vi "Front Panel.vi"(11 "GUI In":refnum<class "Calibration UI.lvclass">) -> ()   [LabVIEW 2015, in "Calibration UI.lvclass"]
uses:
  Calibration UI.lvclass
  Calibration/Collect Data/Collect Data.lvclass
  Calibration/Get Max Orf Flow/Get Max Orifice Flow.lvclass
  Calibration/Set QO2 Rel Flow/Set Rel QO2 flow.lvclass
  Calibration/Set QO2 Rel Flow/Set Rel QO2 flow.lvclass/Set Rel QO2 flow.ctl
  Calibration/Get Max Orf Flow/Get Max Orifice Flow.lvclass/Get Max Orifice Flow.ctl
  Reusable/GUI/GUI.lvclass/GUI.ctl
  Calibration UI.lvclass/Calibration UI.ctl
  Calibration/Collect Data/Collect Data.lvclass/Collect Data.ctl
  Reusable/Sequence/SEQ/SEQ.lvclass
  Reusable/Sequence/STEPS/STEP.lvclass
  Calibration/O3 Generator State/Change O3 Generator State.lvclass
  Calibration/Change Filter State/Change Filter Position.lvclass
  Calibration/Change O2 Valve.lvclass
  Calibration/Wait/Wait.lvclass
  Calibration/Wait/Wait.lvclass/Wait.ctl
  Reusable/Sequence/STEPS/LEAVES/Double/Switch DBL.lvclass/Switch DBL.ctl
  Calibration/O3 Add Valve/Ozone Addition Valve.lvclass
  Calibration/Set O3 Level/Set O3 Level.lvclass
  Calibration/Set O3 Level/Set O3 Level.lvclass/Set O3 Level.ctl
  Calibration/Change Spk Pos/Change Speaker Position.lvclass
  Calibration/State data/State Data.lvclass
  Controls/MFC Address.ctl
  Controls/Flags.ctl
  Reusable/GUI/Accessors/Read RegEvent.vi
  Calibration/Wait/Write Wait Time.vi
  Reusable/Sequence/STEPS/LEAVES/Double/Write val.vi
  Calibration/Collect Data/Write # of Obs.vi
  Calibration/Collect Data/Write Stored State DVR.vi
  Calibration/Collect Data/Write PAS DVR.vi
  Calibration/Collect Data/Write CRD DVR.vi
  Calibration/Collect Data/Write Associated Cells.vi
  Calibration/Set QO2 Rel Flow/Write QO2 DVR.vi
  Calibration/Get Max Orf Flow/Write Max Qorf DVR.vi
panel:
  in  "Lamp":bool
  in  "Lamp Rate (Hz)":i32
  in  "cSequence":bool
  in  "lSequence":bool
  in  "cTable":bool
  out "collPoints":i32
  in  "saveSeq":bool
  in  "Steps":string(tree)
  in  "Sequence":string(tree)
  in  "setCal":bool caption="Set Calibration\nParameters"
  in  "Display":T1(ring)
  in  "O2 Flow":sgl caption="O2 Flow\n(sccm)" format="%.2g"
  in  "Valves":cluster{"O3 Add":bool, "O2 Open":bool}
  out "O3Q":cluster{"Q":sgl, "T":sgl, "P":sgl} caption="Alicat Data" {"P" format="%.2f"; "T" format="%.2f"; "Q" format="%.2f"}
  out "r^2":dbl
  out "Intercept":dbl
  out "Slope":dbl
  out "cal Results":cluster{dbl[], "Upper Bound":dbl[]}[](graph)
  in  "calibrate":bool caption="Run Calibration"
  out "seqMsg":string[](array[string])=["1:09:27 PM\tValve to oxygen changed to TRUE.", "1:09:27 PM\tO2 flow set to 500.000000.", "1:09:32 PM\tMax orifice flow recorded.   Flow was 248.806366.", "1:09:42 PM\tStandard wait time elapsed.", "1:09:54 PM\tStandard wait time elapsed.", "1:09:55 PM\tLaser RMS stable in every cell. RSE Values: 0.000000\t0.000000\r\n", "1:09:55 PM\tSpeaker position changed to TRUE.", "1:09:55 PM\tO2 flow set to 248.806366.", "1:10:01 PM\tOzone stable in every cell.  Begin collecting data. RSE Values: 0.043430\t0.043108\t0.043108\t0.043537\t0.043537\t0.047428\t0.047428\t0.043882\t0.043882\t0.044978\t0.044978\t0.043616\t0.043616\t0.042956\r\n", "1:10:21 PM\tCollection step complete.", "1:10:21 PM\tO2 flow set to 186.604774.", "1:10:27 PM\tOzone stable in every cell.  Begin collecting data. RSE Values: 0.049616\t0.048562\t0.048562\t0.048143\t0.048143\t0.048496\t0.048678\t0.048678\t0.047656\t0.047656\t0.046716\t0.046716\t0.046716\r\n", "1:10:47 PM\tCollection step complete.", "1:10:47 PM\tO2 flow set to 124.403183.", "1:10:53 PM\tOzone stable in every cell.  Begin collecting data. RSE Values: 0.045074\t0.045269\t0.045269\t0.045371\t0.045371\t0.046657\t0.046657\t0.044803\t0.044803\t0.046626\t0.046626\t0.044248\t0.044248\t0.044248\r\n", "1:11:13 PM\tCollection step complete.", "1:11:13 PM\tO2 flow set to 62.201591.", "1:11:19 PM\tOzone stable in every cell.  Begin collecting data. RSE Values: 0.047075\t0.046939\t0.046939\t0.049594\t0.049594\t0.046739\t0.046655\t0.046655\t0.046655\t0.048990\t0.048989\t0.048989\t0.048989\r\n", "1:11:39 PM\tCollection step complete.", "1:11:39 PM\tData displayed!", "1:11:39 PM\tSpeaker position changed to FALSE.", "1:11:39 PM\tValve to oxygen changed to FALSE.", "1:11:39 PM\tO2 flow set to 0.000000.", "1:11:49 PM\tStandard wait time elapsed.", "1:12:02 PM\tStandard wait time elapsed."] caption="Messages"
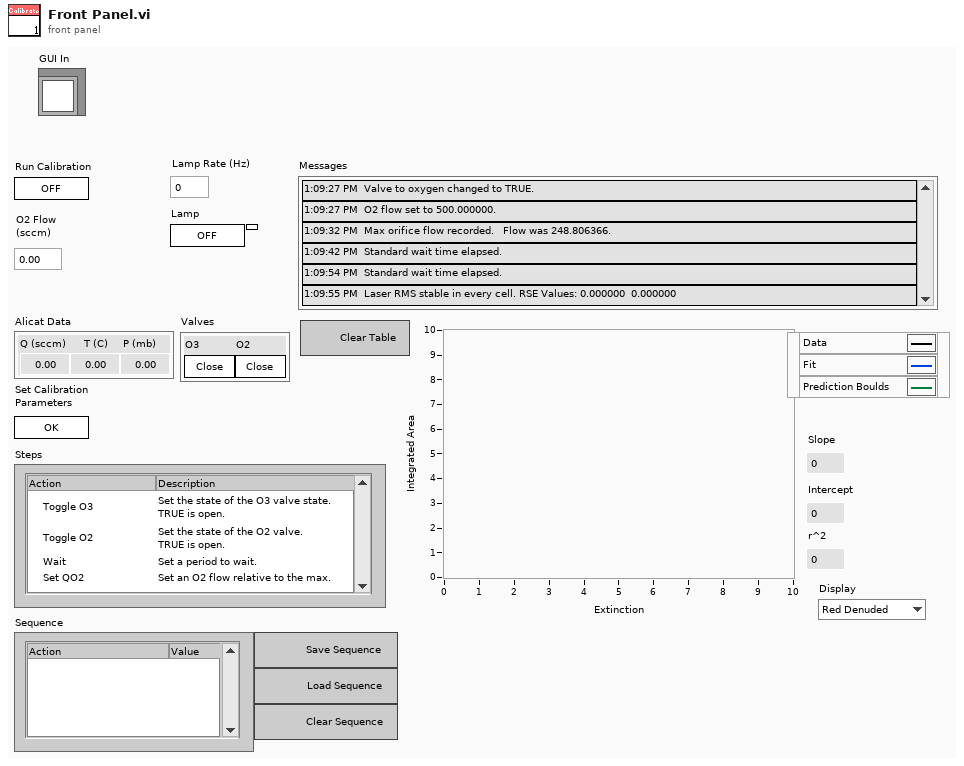
[diagram p1: front panel]
types:
  T1 = enum16{"Red Denuded", "Green", "Red", "Blue", "Blue Denuded"}
  T2 = enum8{"Enabled", "Disabled", "Disabled and Grayed Out"}
  T3 = cluster{"Array of Boolean[0]":bool, "Array of Boolean[1]":bool}
  T4 = cluster{"slope":dbl, "intercept":dbl, "r^2":dbl}[]
  T5 = typedef "Flags.ctl" = enum8{"Autospeaker", "Link cycles", "Autofilter", "O3 Cal", "Filter Position"}
  T6 = typedef "MFC Address.ctl" = enum16{"CRDS Purge", "CRDS Thermodenuded", "CRDS Dry", "CRDS Med RH", "CRDS High RH", "PAS Ch 1", "PAS Ch 2", "PAS Ch3", "PAS Ch 4", "PAS Ch 5", "CLAP", "O3", "Pinlet"}
  T7 = cluster{"Numeric":sgl, "Numeric":sgl, "Numeric":sgl}
  T8 = typedef "eventvkey.ctl" = enum16{"ASCII", "Enter", "Return", "Shift", "Ctrl", "Alt", "Cmd", "Opt", "Caps", "NumLock", "Clear", "Break", "Up", "Down", "Left", "Right", "Insert", "Delete", "Home", "End", "PageUp", "PageDown", "Escape", "Help", "Pause", "ScrollLock", "F1", "F2", "F3", "F4", "F5", "F6", "F7", "F8", "F9", "F10", "F11", "F12", "F13", "F14", "F15", "F16", "F17", "F18", "F19", "F20", "F21", "F22", "F23", "F24", "Play", "VolumeUp", "VolumeDown", "Mute", "Two Byte Char"}
  T9 = cluster{"Stored State":refnum<class "State Data.lvclass">[], "pointer to data":i32}
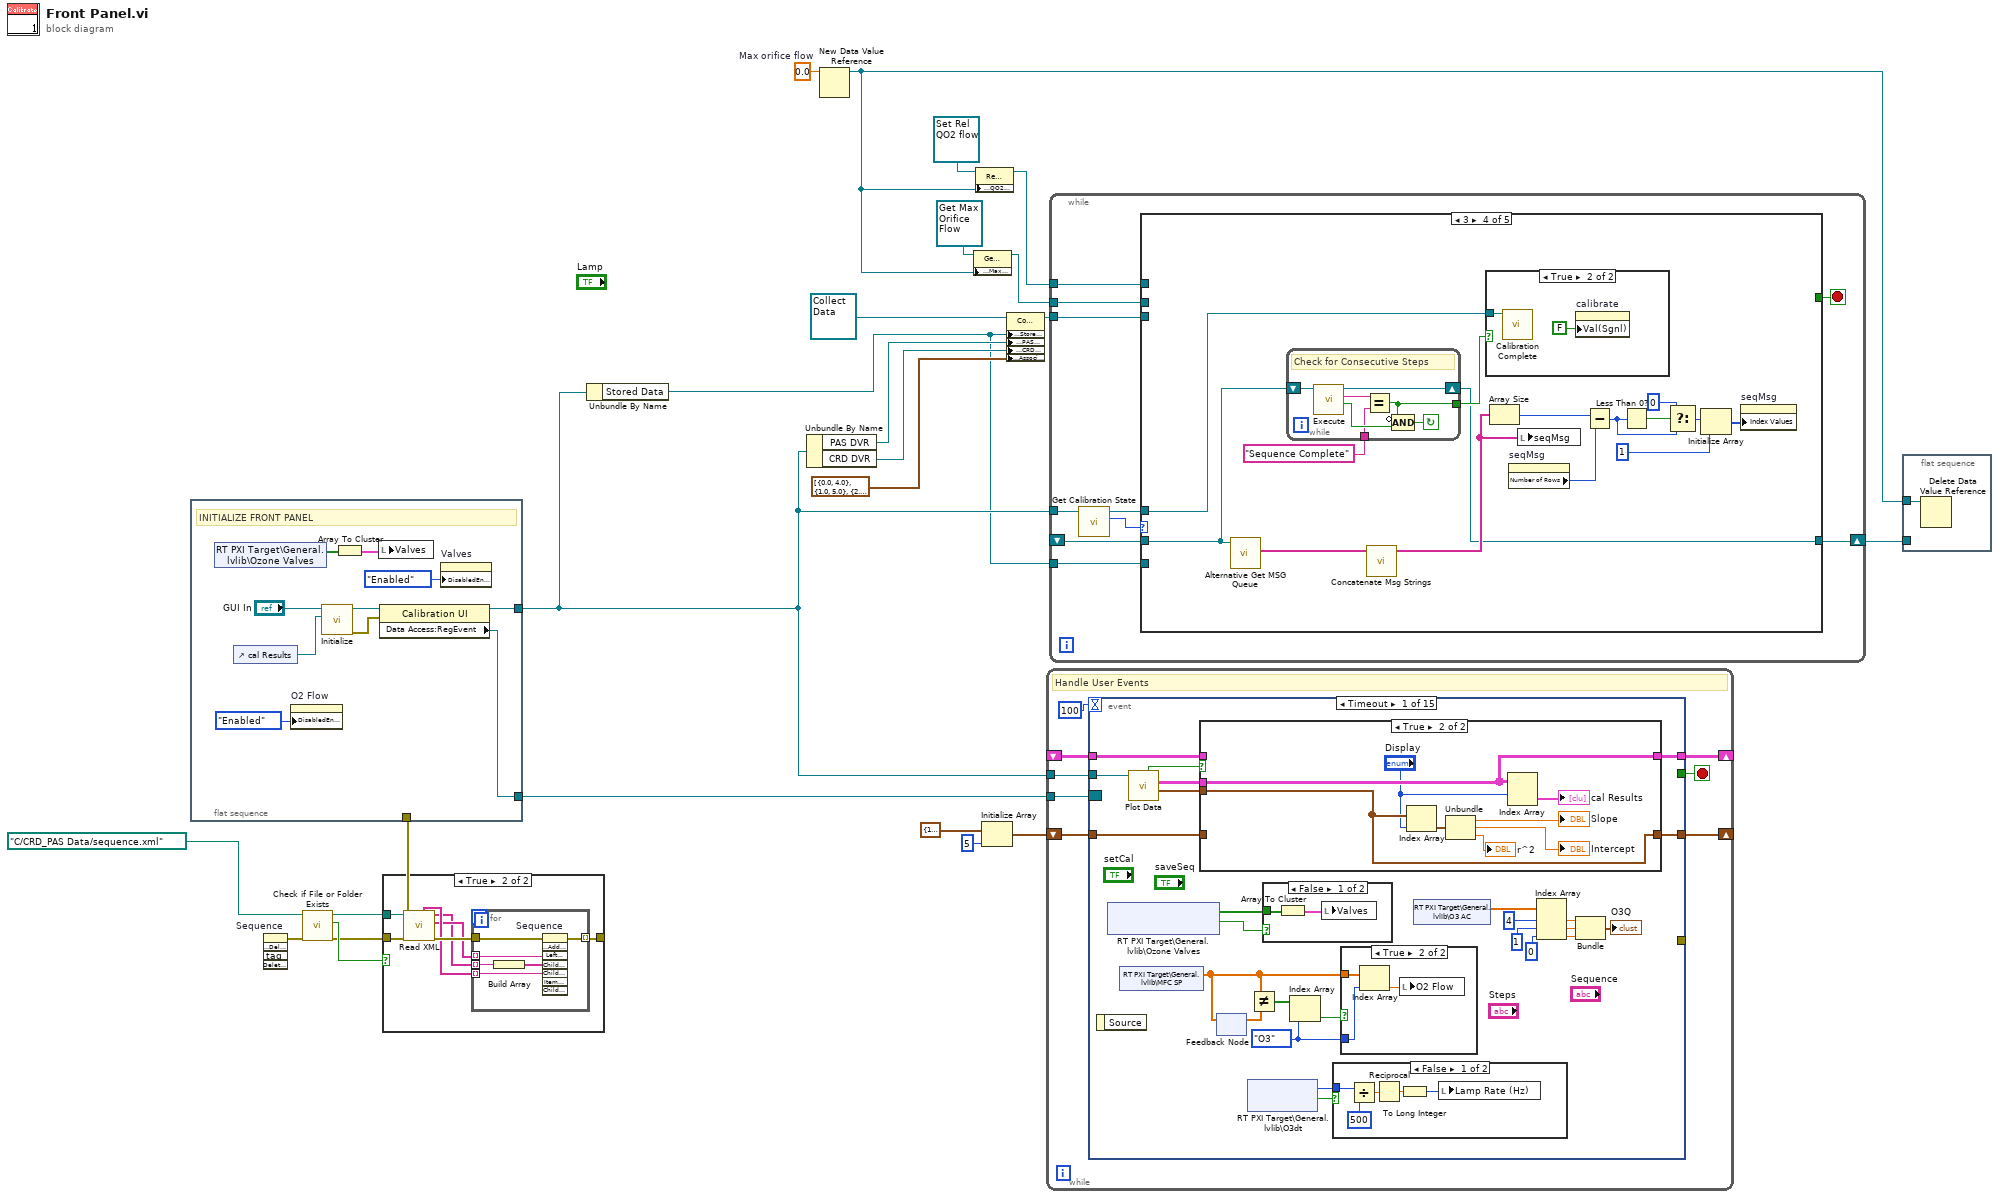
[diagram p0: block diagram]
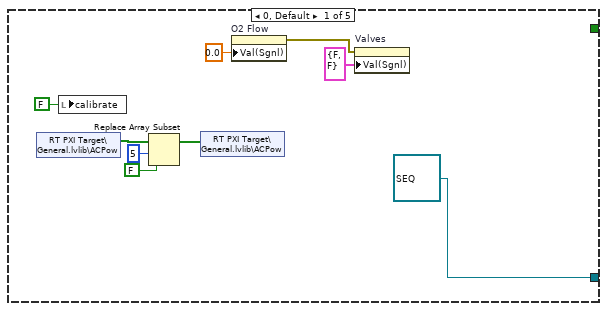
[diagram p3: hidden frame]
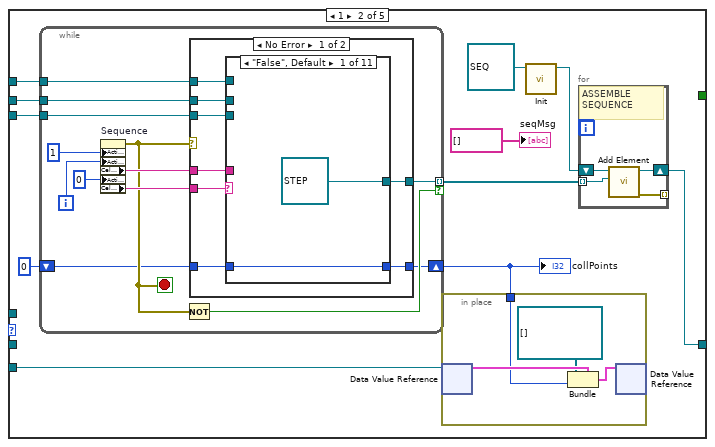
[diagram p4: hidden frame]
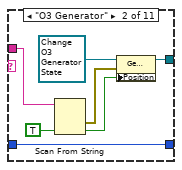
[diagram p5: hidden frame]
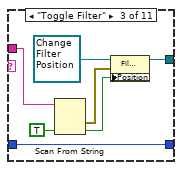
[diagram p6: hidden frame]
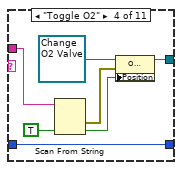
[diagram p7: hidden frame]
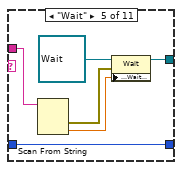
[diagram p8: hidden frame]
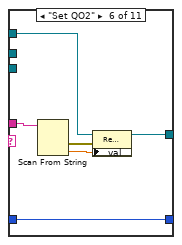
[diagram p9: hidden frame]
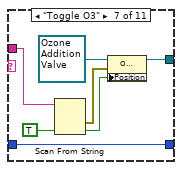
[diagram p10: hidden frame]
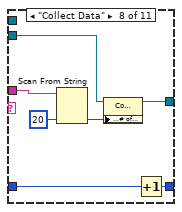
[diagram p11: hidden frame]
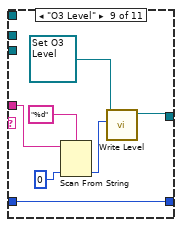
[diagram p12: hidden frame]
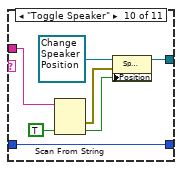
[diagram p13: hidden frame]
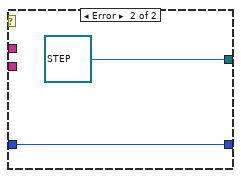
[diagram p15: hidden frame]
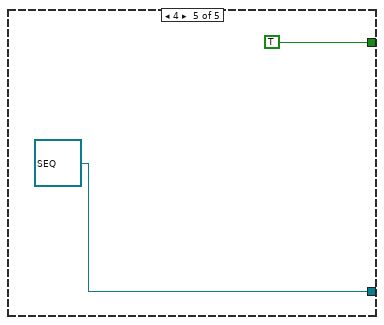
[diagram p18: hidden frame]
diagram:
  w20 = 0.0  # Max orifice flow
  n1 = flat-sequence {
    tunnel: [w27] -> w24
    tunnel: [w26] -> w2
    tunnel: w6 -> [_]
    frame #0 {
      # "INITIALIZE FRONT PANEL"
      n2 = shared-variable "RT PXI Target\\General.lvlib\\Ozone Valves"() -> (w34:bool[])  [unwired: 1 in, 1 out]
      n3 = control-ref of="cal Results"() -> (w30:refnum<vi>)
      n4 = property on="O2 Flow" class="DigNum (strict)"("DisabledEnum"=T2."Enabled" ("Disabled")) -> ()  [unwired: 2 in, 2 out]
      n5 = call "Initialize.vi"("XYGraph in"=w30, "GUI In"="GUI In") -> ("error out"=w29:errorcluster, "GUI Out"=w31:refnum<class "Calibration UI.lvclass">)  [unwired: 8 in]
      n6 = Array To Cluster(array=w34) -> (cluster=w33:T3)
      n7 = local write "Valves"(w33) -> ()
      n8 = property class="Calibration UI"(reference=w31, error in=w29) -> (reference out=w26:refnum<class "Calibration UI.lvclass">, "Data Access:RegEvent"=w27:refnum<event-registration>)  [unwired: 1 out]
      n9 = property on="Valves" class="Clust (strict)"("DisabledEnum"=T2."Enabled" ("Disabled")) -> ()  [unwired: 2 in, 2 out]
    }
  }
  n10 = invoke on="Sequence" class="Tree (strict)" method="Edit Tree Items.Delete"() -> (error out=w9:errorcluster)  [unwired: 5 in, 4 out]
  n11 = call <vilib>:"Check if File or Folder Exists.vi"("error in (no error)"=w9, "path"=path "C:/CRD_PAS Data/sequence.xml" ("file")) -> ("error out"=w8:errorcluster, "file or folder exists?"=w10:bool, "dup path"=w7:path)  [unwired: 7 in]
  n12 = case shown="True" w10 {
    tunnel: w8 -> [_ w37]
    tunnel: w7 -> [_ w39]
    tunnel: [_ w35] -> w6
    frame False {
    }
    frame True {
      n13 = call "Read XML.vi"("error in"=w37, "path"=w39) -> ("error out"=w36:errorcluster, "Steps"=w40:string[], "Values"=w38:string[], "tags"=w41:string[])  [unwired: 5 in, 1 out]
      n14 = for {
        tunnel: w41 -> [w47] mode=indexing
        tunnel: w40 -> [w46] mode=indexing
        tunnel: w38 -> [w45] mode=indexing
        tunnel: w36 -> [w43]
        tunnel: [w42] -> w35 mode=indexing
        n15 = Build Array(w45) -> (w44:string[])
        n16 = invoke on="Sequence" class="Tree (strict)" method="Edit Tree Items.Add Item to End"(error in=w43, "Left Cell"=w46, "Child Text"=w44, "Child Tag"=w47) -> (error out=w42:errorcluster)  [unwired: 4 in, 7 out]
      }
    }
  }
  n17 = Unbundle By Name(w2) -> ("Stored Data"=w1:refnum<data-value>)
  n18 = Unbundle By Name(w2) -> ("PAS DVR"=w17:refnum<data-value>, "CRD DVR"=w16:refnum<data-value>)
  n19 = New Data Value Reference(data value=w20) -> (data value reference=w4:refnum<data-value>)  [unwired: 1 in, 1 out]
  n20 = property class="Get Orifice Qmax"(reference=refnum<class "Get Max Orifice Flow.lvclass"> refnum ("Get Orifice Qmax"), "Data Access:Max Qorf DVR"=w4) -> (reference out=w12:refnum<class "Get Max Orifice Flow.lvclass">)  [unwired: 1 in, 1 out]
  n21 = property class="Rel O2 Flow"(reference=refnum<class "Set Rel QO2 flow.lvclass"> refnum ("Rel O2 Flow"), "Data Access:QO2 DVR"=w4) -> (reference out=w3:refnum<class "Set Rel QO2 flow.lvclass">)  [unwired: 1 in, 1 out]
  n22 = Initialize Array(cluster{"slope":dbl, "intercept":dbl, "r^2":dbl} {"slope"=1.0, "intercept"=0.0, "r^2"=0.0} ("Linear Fit Data"), 5 ("dimension size")) -> (w21:T4)
  n23 = property class="Collect Data.lvclass"(reference=refnum<class "Collect Data.lvclass"> refnum ("Collect Data.lvclass"), "Data Access:Stored State DVR"=w1, "Data Access:PAS DVR"=w17, "Data Access:CRD DVR"=w16, "Data Access:Associated Cells"=cluster{"PAS":dbl, "CRD":dbl}[] [{"PAS"=0.0, "CRD"=4.0}, {"PAS"=1.0, "CRD"=5.0}, {"PAS"=2.0, "CRD"=4.0}, {"PAS"=3.0, "CRD"=3.0}, {"PAS"=4.0, "CRD"=3.0}] ("Associated Cells")) -> (reference out=w15:refnum<class "Collect Data.lvclass">)  [unwired: 1 in, 1 out]
  n24 = while {
    tunnel: w24 -> [w55]
    tunnel: w2 -> [w52]
    shift-right: [w51] -> _
    shift-left: _ -> [w50]
    shift-right: [w49] -> _
    shift-left: w21 -> [w48]
    stop <- w54 stop-if-true
    # "Handle User Events"
    n25 = event shown="[0] Timeout" {
      selector: w55 -> [_ _ _ _ _ _ _ _ _ _ _ _ _ _ _]
      dyn-events: _ -> [_ _ _ _ _ _ _ _ _ _ _ _ _ _ _]
      timeout: 100 -> [_ _ _ _ _ _ _ _ _ _ _ _ _ _ _]
      tunnel: [_ _ _ _ _ _ _ _ _ _ _ _ _ TRUE _] -> w54
      tunnel: w52 -> [w72 _ _ _ _ _ _ w201 _ _ _ _ _ w256 _]
      tunnel: [w68 w103 w110 w123 w130 w134 w157 w197 w216 w228 w242 w244 w252 w255 w264] -> w51
      tunnel: w50 -> [w67 w103 w110 w123 w130 w134 w157 w197 w216 w228 w242 w244 w252 w255 w264]
      tunnel: [w66 w102 w109 w115 w129 w133 w158 w196 w215 w227 w229 w243 w251 w254 w263] -> w49
      tunnel: w48 -> [w65 w102 w109 w115 w129 w133 w158 w196 w215 w227 w229 w243 w251 w254 w263]
      tunnel: [_ _ _ _ _ _ _ _ w210 _ _ _ _ _ _] -> _
      event Timeout {
        w59 = MFC_Address."O3" ("Controllers")
        n26 = event-data() -> ()  [unwired: 1 in, 1 out]
        n27 = shared-variable "RT PXI Target\\General.lvlib\\Ozone Valves"() -> (w58:bool[], w64:bool)  [unwired: 2 in, 1 out]
        n28 = shared-variable "RT PXI Target\\General.lvlib\\MFC SP"() -> (w60:sgl[])  [unwired: 1 in, 1 out]
        n29 = call "Plot Data.vi"("GUI In"=w72) -> ("Fit Data"=w69:T4, "Plot Data"=w70:cluster{dbl[], "Upper Bound":dbl[]}[][], "Data Available?"=w71:bool)  [unwired: 7 in, 1 out]
        n30 = case shown="True" w71 {
          tunnel: w70 -> [_ w99]
          tunnel: w69 -> [_ w94]
          tunnel: [w92 w99] -> w68
          tunnel: w67 -> [w92 _]
          tunnel: [w91 w94] -> w66
          tunnel: w65 -> [w91 _]
          frame False {
          }
          frame True {
            n31 = Index Array(array=w94, index="Display") -> (element=w98:cluster{"slope":dbl, "intercept":dbl, "r^2":dbl})
            n32 = Unbundle(w98) -> ("slope"=→"Slope":dbl, "intercept"=→"Intercept":dbl, "r^2"=→"r^2":dbl)
            n33 = Index Array(array=w99, index (row)="Display") -> (element=→"cal Results":cluster{dbl[], "Upper Bound":dbl[]}[])  [unwired: 1 in]
          }
        }
        n34 = feedback #1() -> (w63:sgl[])  [unwired: 1 in]
        n35 = feedback-in #1(w60) -> ()
        n36 = shared-variable "RT PXI Target\\General.lvlib\\O3dt"() -> (w56:i64, w57:bool)  [unwired: 2 in, 1 out]
        n37 = Not Equal?(x=w60, y=w63) -> (x != y?=w62:bool[])
        n38 = case shown="False" w64 {
          tunnel: w58 -> [w89 _]
          frame False {
            n39 = Array To Cluster(array=w89) -> (cluster=w90:T3)
            n40 = local write "Valves"(w90) -> ()
          }
          frame True {
          }
        }
        n41 = Index Array(array=w62, index=w59) -> (element=w61:bool)
        n42 = case shown="False" w57 {
          tunnel: w56 -> [w85 _]
          frame False {
            n43 = Divide(x=w85, y=i64 500) -> (x/y=w83:dbl)
            n44 = Reciprocal(x=w83) -> (1/x=w82:dbl)
            n45 = To Long Integer(number=w82) -> (32bit integer=w81:i32)
            n46 = local write "Lamp Rate (Hz)"(w81) -> ()
          }
          frame True {
          }
        }
        n47 = case shown="True" w61 {
          tunnel: w60 -> [_ w88]
          tunnel: w59 -> [_ w87]
          frame False {
          }
          frame True {
            n48 = Index Array(array=w88, index=w87) -> (element=w86:sgl)
            n49 = local write "O2 Flow"(w86) -> ()
          }
        }
        n50 = shared-variable "RT PXI Target\\General.lvlib\\O3 AC"() -> (w80:sgl[])  [unwired: 1 in, 1 out]
        n51 = Index Array(array=w80, index #1=4 ("index"), index #2=1 ("index"), index #3=0 ("index")) -> (element #1=w76:sgl, element #2=w75:sgl, element #3=w74:sgl)
        n52 = Bundle("Numeric"=w76, "Numeric"=w75, "Numeric"=w74) -> (→"O3Q":T7)  [unwired: 1 in]
      }
      event "Lamp Rate (Hz)": Value Change {
        n53 = event-data() -> ()  [unwired: 1 in, 3 out]
        n54 = To Double Precision Float(number="Lamp Rate (Hz)") -> (double precision float=w106:dbl)
        n55 = Reciprocal(x=w106) -> (1/x=w101:dbl)
        n56 = Multiply(x=w101, y=500.0) -> (x*y=w105:dbl)
        n57 = To Quad Integer(1:w105) -> (0:w104:i64)
        n58 = shared-variable "RT PXI Target\\General.lvlib\\O3dt"(w104) -> ()  [unwired: 1 in, 1 out]
      }
      event "Sequence": Key Down {
        n59 = event-data() -> ("VKey"=w111:T8)  [unwired: 1 in]
        n60 = case shown="\"Delete\"" w111 {
          frame "ASCII", Default {
          }
          frame "Delete" {
            n61 = local read "Sequence"() -> (w113:string)
            n62 = invoke on="Sequence" class="Tree (strict)" method="Edit Tree Items.Delete"("tag"=w113, "Delete Children"=TRUE ("Delete Children?")) -> ()  [unwired: 3 in, 5 out]
          }
        }
      }
      event "Steps": Double Click {
        n63 = event-data() -> ("Tag"=w114:string)  [unwired: 1 in]
        n64 = property on="Steps" class="Tree (strict)"("Active Item Tag"=w114, "ActiveColNum"=0 ("Active Cell:Active Column Number")) -> ("Cell String"=w121:string, "Active Item Tag"=w116:string)  [unwired: 2 in, 2 out]
        n65 = Match Pattern(string=w116, regular expression=":" ("search string/char (-)")) -> (before substring=w117:string)  [unwired: 1 in, 3 out]
        n66 = case shown="\"U16\"" w117 {
          tunnel: [string[] [] w125 string[] ["0"] string[] ["20"]] -> w119
          frame "False", Default {
          }
          frame "bool" {
            n67 = Build Array("TRUE") -> (w125:string[])
          }
          frame "U8", "dbl" {
          }
          frame "U16" {
          }
        }
        n68 = invoke on="Sequence" class="Tree (strict)" method="Edit Tree Items.Add Item to End"("Left Cell"=w121, "Child Text"=w119, "Child Tag"=w116, "Item Indent"=0 ("New Item Indentation")) -> ()  [unwired: 4 in, 8 out]
      }
      event "cSequence": Value Change {
        n69 = event-data() -> ()  [unwired: 1 in, 1 out]
        n70 = invoke on="Sequence" class="Tree (strict)" method="Edit Tree Items.Delete"() -> ()  [unwired: 5 in, 5 out]
      }
      event "lSequence": Value Change {
        n71 = event-data() -> ()  [unwired: 1 in, 6 out]
        n72 = call "File Dialog"("prompt"="Open sequence file.", "pattern (all files)"="*.xml") -> ("selected path"=w136:path, "cancelled"=w132:bool, "error out"=w131:errorcluster)  [unwired: 10 in, 1 out]
        n73 = case shown="False" w132 {
          tunnel: w136 -> [w143 _]
          tunnel: [w140 _] -> _
          tunnel: w131 -> [w139 _]
          frame False {
            n74 = invoke on="Sequence" class="Tree (strict)" method="Edit Tree Items.Delete"(error in=w139) -> (error out=w138:errorcluster)  [unwired: 4 in, 4 out]
            n75 = call "Read XML.vi"("error in"=w138, "path"=w143) -> ("error out"=w141:errorcluster, "Steps"=w144:string[], "Values"=w142:string[], "tags"=w145:string[])  [unwired: 5 in, 1 out]
            n76 = for {
              tunnel: w145 -> [w151] mode=indexing
              tunnel: w144 -> [w150] mode=indexing
              tunnel: w142 -> [w149] mode=indexing
              tunnel: w141 -> [w147]
              tunnel: [w146] -> w140 mode=indexing
              n77 = Build Array(w149) -> (w148:string[])
              n78 = invoke on="Sequence" class="Tree (strict)" method="Edit Tree Items.Add Item to End"(error in=w147, "Left Cell"=w150, "Child Text"=w148, "Child Tag"=w151) -> (error out=w146:errorcluster)  [unwired: 4 in, 7 out]
            }
          }
          frame True {
          }
        }
      }
      event "Sequence": Edit Cell? {
        n79 = event-data() -> ("Tag"=w154:string, "String"=w153:string)  [unwired: 1 in]
        n80 = Match Pattern(string=w154, regular expression=":" ("search string/char (-)")) -> (before substring=w155:string)  [unwired: 1 in, 3 out]
        n81 = case shown="\"bool\"" w155 {
          tunnel: w153 -> [w159 w163 w176 w178]
          tunnel: [w159 w160 w169 w177] -> w152
          frame "", Default {
          }
          frame "bool" {
            w161 = "FALSE" ("x")
            n82 = Not Equal?(x=w163, y="TRUE") -> (x != y?=w165:bool)
            n83 = Not Equal?(x=w161, y=w163) -> (x != y?=w164:bool)
            n84 = And(x=w164, y=w165) -> (x .and. y?=w162:bool)
            n85 = case shown="False" w162 {
              tunnel: w163 -> [w167 _]
              tunnel: [w167 w168] -> w160
              tunnel: w161 -> [_ w168]
              frame False {
              }
              frame True {
              }
            }
          }
          frame "U8" {
            n86 = Scan From String(format string="%d", input string=w176, default 1=u8 0 ("default value 1")) -> (output 1=w173:u8)  [unwired: 2 in, 3 out]
            n87 = In Range and Coerce(upper limit=u8 15, x=w173, lower limit=u8 0) -> (coerced(x)=w170:u8)  [unwired: 1 out]
            n88 = Format Into String(w170) -> (resulting string=w169:string)  [unwired: 3 in, 1 out]
          }
          frame "dbl" {
            n89 = Scan From String(input string=w178, default 1=0.0 ("default value 1")) -> (error out=w179:errorcluster)  [unwired: 4 in, 2 out]
            n90 = case shown="No Error" w179 {
              tunnel: w178 -> [w181 _]
              tunnel: [w181 "0" ("NewVal")] -> w177
              frame No Error {
              }
              frame Error {
              }
            }
          }
        }
        n91 = event-data("String"=w152) -> ()  [unwired: 1 in, 1 out]
      }
      event "calibrate": Value Change {
        w190 = u8 1 ("Plot.Line Width")
        n92 = event-data() -> ()  [unwired: 1 in, 1 out]
        n93 = call "Change Calibration State.vi"("New State"="calibrate", "Calibration UI in"=w201) -> ()  [unwired: 8 in, 2 out]
        n94 = control-ref of="cal Results"() -> (w194:refnum<vi>)
        n95 = local read "collPoints"() -> (w195:i32)
        n96 = Select(t=T2."Disabled and Grayed Out" ("Disabled"), s="calibrate", f=T2."Enabled") -> (s? t:f=w198:T2)
        n97 = shared-variable "RT PXI Target\\General.lvlib\\O3On"("calibrate") -> ()  [unwired: 1 in, 1 out]
        n98 = Subtract(x=w195, y=4) -> (x-y=w192:i32)
        n99 = shared-variable "RT PXI Target\\General.lvlib\\flags"() -> (w189:u8)  [unwired: 1 in, 1 out]
        n100 = for {
          N: w192 -> [_]
          tunnel: w194 -> [w209]
          tunnel: u32 0 -> [w206]
          tunnel: w190 -> [w205]
          tunnel: w190 -> [w204]
          i -> [w208]
          # "HANDLE ERROR BARS"
          n101 = Add(x=w208, y=4) -> (x+y=w203:i32)
          n102 = To Unsigned Long Integer(number=w203) -> (unsigned 32bit integer=w202:u32)
          n103 = property class="XYGraph (strict)"(reference=w209, "Active Plot"=w202, "Plot.Line Style"=w204, "Plot.Line Width"=w205, "Plot.Plot Color"=w206) -> ()  [unwired: 1 in, 2 out]
        }
        n104 = Number To Boolean Array(number=w189) -> (Boolean array=w188:bool[])
        n105 = Replace Array Subset(array=w188, new element="calibrate", index=Flags."O3 Cal" ("Flags")) -> (w187:bool[])
        n106 = property on="O2 Flow" class="DigNum (strict)"("DisabledEnum"=w198) -> ()  [unwired: 2 in, 2 out]
        n107 = Boolean Array To Number(Boolean array=w187) -> (number=w186:u32)
        n108 = To Unsigned Byte Integer(number=w186) -> (unsigned 8bit integer=w185:u8)
        n109 = property on="Valves" class="Clust (strict)"("DisabledEnum"=w198) -> ()  [unwired: 2 in, 2 out]
        n110 = shared-variable "RT PXI Target\\General.lvlib\\flags"(w185) -> ()  [unwired: 1 in, 1 out]
      }
      event "saveSeq": Value Change {
        n111 = event-data() -> ()  [unwired: 1 in, 1 out]
        n112 = while {
          tunnel: [w221] -> w213 mode=indexing if=w222
          tunnel: [w218] -> w212 mode=indexing if=w222
          tunnel: [w217] -> w211 mode=indexing if=w222
          i -> [w220]
          stop <- w224 stop-if-true
          n113 = property on="Sequence" class="Tree (strict)"("Active Item Row Number"=w220, "ActiveColNum"=0 ("Active Cell:Active Column Number"), "ActiveColNum"=1 ("Active Cell:Active Column Number")) -> (error out=w224:errorcluster, "Active Item Tag"=w221:string, "Cell String"=w218:string, "Cell String"=w217:string)  [unwired: 2 in, 1 out]
          n114 = Unbundle By Name(w224) -> ("status"=w225:bool)
          n115 = Not(x=w225) -> (.not. x?=w222:bool)
        }
        n116 = call "Convert Tree Data and Save to XML.vi"("tag"=w213, "Value"=w211, "Step"=w212, "file"=path "C:/CRD_PAS Data/sequence.xml") -> ("error out"=w210:errorcluster)  [unwired: 5 in, 2 out]
      }
      event "cTable": Value Change {
        n117 = event-data() -> ()  [unwired: 1 in, 1 out]
        n118 = local write "seqMsg"(string[] [] ("seqMsg")) -> ()
      }
      event "setCal": Value Change {
        n119 = event-data() -> ()  [unwired: 1 in, 1 out]
        n120 = Current VI's Path() -> (path=w240:path)
        n121 = Strip Path(path=w240) -> (stripped path=w239:path)  [unwired: 1 out]
        n122 = Build Path(base path=w239, name or relative path="Display Calibration Results.vi") -> (appended path=w237:path)
        n123 = Open VI Reference(type specifier VI Refnum (for type only)=refnum<vi> refnum, vi path=w237, options=128) -> (vi reference=w233:refnum<vi>, error out=w231:errorcluster)  [unwired: 3 in]
        n124 = invoke class="VI (strict)" method="FP.Open"(reference=w233, error in=w231) -> (reference out=w232:refnum<vi>, error out=w230:errorcluster)  [unwired: 3 in, 3 out]
        n125 = call-by-ref "Start Asynchronous Call"(reference=w232, error in=w230, "Fit Data"=w229) -> (reference out=w235:refnum<vi>, error out=w234:errorcluster)  [unwired: 11 in]
        n126 = Close Reference(reference=w235, error in (no error)=w234) -> ()  [unwired: 1 out]
      }
      event "O2 Flow": Value Change {
        n127 = event-data() -> ()  [unwired: 1 in, 1 out]
        n128 = shared-variable "RT PXI Target\\General.lvlib\\MFC SP"() -> (w248:sgl[])  [unwired: 1 in, 1 out]
        n129 = in-place {
          in-place-border: "O2 Flow" -> [w249]
          n130 = in-place-array #2(w248, MFC_Address."O3" ("Controllers")) -> ()  [unwired: 1 out]
          n131 = in-place-array #2(w249) -> (w247:sgl[])  [unwired: 1 out]
        }
        n132 = shared-variable "RT PXI Target\\General.lvlib\\MFC SP"(w247) -> ()  [unwired: 1 in, 1 out]
      }
      event "Valves": Value Change {
        n133 = event-data() -> ("NewVal"=w253:cluster{"O3 Add":bool, "O2 Open":bool})  [unwired: 1 in]
        n134 = Cluster To Array(cluster=w253) -> (array=w250:bool[])
        n135 = shared-variable "RT PXI Target\\General.lvlib\\Ozone Valves"(w250) -> ()  [unwired: 1 in, 1 out]
      }
      event User Event; Panel Close {
        n136 = event-data() -> ()  [unwired: 1 in, 1 out]
        n137 = call-dynamic "Stop FP.vi"("Calibration UI in"=w256) -> ()  [unwired: 9 in, 2 out]
      }
      event "Display": Value Change {
        n138 = event-data() -> ("NewVal"=w262:T1)  [unwired: 1 in]
        n139 = Index Array(array=w264, index (row)=w262) -> (element=w265:cluster{dbl[], "Upper Bound":dbl[]}[])  [unwired: 1 in]
        n140 = Index Array(array=w263, index=w262) -> (element=w261:cluster{"slope":dbl, "intercept":dbl, "r^2":dbl})
        n141 = local write "cal Results"(w265) -> ()
        n142 = Unbundle(w261) -> ("slope"=w258:dbl, "intercept"=w260:dbl, "r^2"=w259:dbl)
        n143 = local write "Slope"(w258) -> ()
        n144 = local write "Intercept"(w260) -> ()
        n145 = local write "r^2"(w259) -> ()
      }
    }
  }
  n146 = while {
    tunnel: w2 -> [w274]
    tunnel: w15 -> [w275]
    shift-right: [w272] -> w14
    shift-left: _ -> [w271]
    tunnel: w12 -> [w268]
    tunnel: w1 -> [w267]
    tunnel: w3 -> [w266]
    stop <- w269 stop-if-true
    n147 = call "Get Calibration State.vi"("Calibration UI in"=w274) -> ("Action"=w273:u32, "Calibration UI out"=w270:refnum<class "Calibration UI.lvclass">)  [unwired: 8 in, 1 out]
    n148 = case shown="3" w273 {
      tunnel: w275 -> [_ w295 _ _ _]
      tunnel: [refnum<class "SEQ.lvclass"> refnum ("New Sequence") w291 w392 w394 refnum<class "SEQ.lvclass"> refnum ("New Sequence")] -> w272
      tunnel: w271 -> [_ _ w392 w393 _]
      tunnel: w270 -> [_ _ _ w395 _]
      tunnel: [_ _ _ _ TRUE] -> w269
      tunnel: w268 -> [_ w288 _ _ _]
      tunnel: w267 -> [_ w287 _ _ _]
      tunnel: w266 -> [_ w285 _ _ _]
      frame 0, Default {
        n149 = shared-variable "RT PXI Target\\General.lvlib\\ACPow"() -> (w277:bool[])  [unwired: 1 in, 1 out]
        n150 = local write "calibrate"(FALSE ("calibrate")) -> ()
        n151 = Replace Array Subset(array=w277, new element=FALSE ("new element/subarray"), index=5) -> (w280:bool[])
        n152 = shared-variable "RT PXI Target\\General.lvlib\\ACPow"(w280) -> ()  [unwired: 1 in, 1 out]
        n153 = property on="O2 Flow" class="DigNum (strict)"("Val(Sgnl)"=sgl 0.0 ("Value (Signaling)")) -> (error out=w283:errorcluster)  [unwired: 2 in, 1 out]
        n154 = property on="Valves" class="Clust (strict)"(error in=w283, "Val(Sgnl)"=cluster{"O3 Add":bool, "O2 Open":bool} {"O3 Add"=FALSE, "O2 Open"=FALSE} ("Value (Signaling)")) -> ()  [unwired: 1 in, 2 out]
      }
      frame 1 {
        n155 = while {
          tunnel: [w311] -> w292 mode=indexing if=w309
          tunnel: w295 -> [w306]
          shift-right: [w307] -> w286
          shift-left: 0 -> [w308]
          tunnel: w288 -> [w305]
          tunnel: w285 -> [w304]
          i -> [w315]
          stop <- w310 stop-if-true
          n156 = property on="Sequence" class="Tree (strict)"("ActiveColNum"=1 ("Active Cell:Active Column Number"), "Active Item Row Number"=w315, "ActiveColNum"=0 ("Active Cell:Active Column Number")) -> (error out=w310:errorcluster, "Cell String"=w312:string, "Cell String"=w313:string)  [unwired: 2 in, 1 out]
          n157 = Not(x=w310) -> (.not. x?=w309:bool)
          n158 = case shown="No Error" w310 {
            tunnel: w313 -> [w324 _]
            tunnel: w312 -> [w323 _]
            tunnel: [w322 refnum<class "STEP.lvclass"> refnum ("Sequence Composition:STEP.lvclass")] -> w311
            tunnel: w308 -> [w321 w390]
            tunnel: [w320 w390] -> w307
            tunnel: w306 -> [w319 _]
            tunnel: w305 -> [w318 _]
            tunnel: w304 -> [w317 _]
            frame No Error {
              n159 = case shown="\"False\", Default" w324 {
                tunnel: [refnum<class "STEP.lvclass"> refnum ("Sequence Composition:STEP.lvclass") w330 w337 w344 w351 w358 w363 w368 w374 w384 w388] -> w322
                tunnel: w323 -> [_ w328 w335 w342 w349 w356 w361 w371 w378 w382 _]
                tunnel: w321 -> [w325 w327 w334 w341 w348 w355 w360 w373 w380 w381 w389]
                tunnel: [w325 w327 w334 w341 w348 w355 w360 w372 w380 w381 w389] -> w320
                tunnel: w319 -> [_ _ _ _ _ _ _ w367 _ _ _]
                tunnel: w318 -> [_ _ _ _ _ _ _ _ _ _ w388]
                tunnel: w317 -> [_ _ _ _ _ w354 _ _ _ _ _]
                frame "False", Default {
                }
                frame "O3 Generator" {
                  n160 = Scan From String(input string=w328, default 1=TRUE) -> (error out=w329:errorcluster, output 1=w332:bool)  [unwired: 3 in, 2 out]
                  n161 = property class="Gen State"(reference=refnum<class "Change O3 Generator State.lvclass"> refnum ("Gen State"), error in=w329, "Position"=w332) -> (reference out=w330:refnum<class "Change O3 Generator State.lvclass">)  [unwired: 1 out]
                }
                frame "Toggle Filter" {
                  n162 = Scan From String(input string=w335, default 1=TRUE) -> (error out=w336:errorcluster, output 1=w339:bool)  [unwired: 3 in, 2 out]
                  n163 = property class="Filter Position"(reference=refnum<class "Change Filter Position.lvclass"> refnum ("Filter Position"), error in=w336, "Position"=w339) -> (reference out=w337:refnum<class "Change Filter Position.lvclass">)  [unwired: 1 out]
                }
                frame "Toggle O2" {
                  n164 = Scan From String(input string=w342, default 1=TRUE) -> (error out=w343:errorcluster, output 1=w346:bool)  [unwired: 3 in, 2 out]
                  n165 = property class="O2 Valve"(reference=refnum<class "Change O2 Valve.lvclass"> refnum ("O2 Valve"), error in=w343, "Position"=w346) -> (reference out=w344:refnum<class "Change O2 Valve.lvclass">)  [unwired: 1 out]
                }
                frame "Wait" {
                  n166 = Scan From String(input string=w349) -> (error out=w350:errorcluster, output 1=w352:dbl)  [unwired: 4 in, 2 out]
                  n167 = property class="Wait"(reference=refnum<class "Wait.lvclass"> refnum ("Wait"), error in=w350, "Data Access:Wait Time"=w352) -> (reference out=w351:refnum<class "Wait.lvclass">)  [unwired: 1 out]
                }
                frame "Set QO2" {
                  n168 = Scan From String(input string=w356) -> (error out=w357:errorcluster, output 1=w359:dbl)  [unwired: 4 in, 2 out]
                  n169 = property class="Rel O2 Flow"(reference=w354, error in=w357, "val"=w359) -> (reference out=w358:refnum<class "Set Rel QO2 flow.lvclass">)  [unwired: 1 out]
                }
                frame "Toggle O3" {
                  n170 = Scan From String(input string=w361, default 1=TRUE) -> (error out=w362:errorcluster, output 1=w365:bool)  [unwired: 3 in, 2 out]
                  n171 = property class="O3 Add"(reference=refnum<class "Ozone Addition Valve.lvclass"> refnum ("O3 Add"), error in=w362, "Position"=w365) -> (reference out=w363:refnum<class "Ozone Addition Valve.lvclass">)  [unwired: 1 out]
                }
                frame "Collect Data" {
                  n172 = Scan From String(input string=w371, default 1=u16 20 ("default value 1")) -> (output 1=w369:u16)  [unwired: 3 in, 3 out]
                  n173 = property class="Collect Data.lvclass"(reference=w367, "Data Access:# of Obs"=w369) -> (reference out=w368:refnum<class "Collect Data.lvclass">)  [unwired: 1 in, 1 out]
                  n174 = Increment(x=w373) -> (x+1=w372:i32)
                }
                frame "O3 Level" {
                  n175 = Scan From String(format string="%d", input string=w378, default 1=u8 0) -> (output 1=w375:u8)  [unwired: 2 in, 3 out]
                  n176 = call "Write Level.vi"("Level"=w375, "Set O3 Level in"=refnum<class "Set O3 Level.lvclass"> refnum ("O3 Level")) -> ("Set O3 Level out"=w374:refnum<class "Set O3 Level.lvclass">)  [unwired: 8 in, 1 out]
                }
                frame "Toggle Speaker" {
                  n177 = Scan From String(input string=w382, default 1=TRUE) -> (error out=w383:errorcluster, output 1=w385:bool)  [unwired: 3 in, 2 out]
                  n178 = property class="Spk Pos"(reference=refnum<class "Change Speaker Position.lvclass"> refnum ("Spk Pos"), error in=w383, "Position"=w385) -> (reference out=w384:refnum<class "Change Speaker Position.lvclass">)  [unwired: 1 out]
                }
                frame "Get Max QO2" {
                }
              }
            }
            frame Error {
            }
          }
        }
        "collPoints" <- w286
        n179 = in-place {
          in-place-border: w286 -> [w298]
          n180 = in-place-dvr #3(w287) -> (w299:T9)  [unwired: 1 out]
          n181 = Bundle(cluster=w299, "Stored State"=refnum<class "State Data.lvclass">[] [], "pointer to data"=w298) -> (w297:T9)
          n182 = in-place-dvr #3(w297) -> ()  [unwired: 2 out]
        }
        n183 = call-dynamic "Init.vi"("SEQ in"=refnum<class "SEQ.lvclass"> refnum) -> ("SEQ out"=w293:refnum<class "SEQ.lvclass">)  [unwired: 9 in, 1 out]
        n184 = for {
          shift-right: [w303] -> w291
          shift-left: w293 -> [w301]
          tunnel: [w302] -> _ mode=indexing
          tunnel: w292 -> [w300] mode=indexing
          # "ASSEMBLE SEQUENCE"
          n185 = call "Add Element.vi"("STEP"=w300, "SEQ in"=w301) -> ("error out"=w302:errorcluster, "SEQ out"=w303:refnum<class "SEQ.lvclass">)  [unwired: 8 in]
        }
        "seqMsg" <- string[] [] ("seqMsg")
      }
      frame 2 {
      }
      frame 3 {
        n186 = call "Alternative Get MSG Queue.vi"("SEQ in"=w393) -> ("seqMsg"=w398:string[])  [unwired: 8 in, 2 out]
        n187 = while {
          shift-right: [w413] -> w394
          shift-left: w393 -> [w414]
          tunnel: [w410] -> w396
          tunnel: "Sequence Complete" ("t") -> [w408]
          stop <- w411 continue-if-true
          # "Check for Consecutive Steps"
          n188 = call-dynamic "Execute.vi"("SEQ in"=w414) -> ("Next Step?"=w409:bool, "MSG"=w412:string, "SEQ out"=w413:refnum<class "SEQ.lvclass">)  [unwired: 7 in, 1 out]
          n189 = Equal?(x=w412, y=w408) -> (x = y?=w410:bool)
          n190 = Compound Arithmetic op=AND(invert w410, w409) -> (w411:bool)
        }
        n191 = call "Concatenate Msg Strings.vi"("StringsIn"=w398) -> ("StringsOut"=w399:string[])  [unwired: 10 in]
        n192 = case shown="True" w396 {
          tunnel: w395 -> [_ w416]
          frame False {
          }
          frame True {
            n193 = call "Calibration Complete.vi"("Calibration UI in"=w416) -> ()  [unwired: 9 in, 2 out]
            n194 = property on="calibrate" class="Bool (strict)"("Val(Sgnl)"=FALSE ("Value (Signaling)")) -> ()  [unwired: 2 in, 2 out]
          }
        }
        n195 = Array Size(array=w399) -> (size(s)=w405:i32)
        n196 = property on="seqMsg" class="Arr (strict)"() -> ("Number of Rows"=w406:u32)  [unwired: 2 in, 2 out]
        n197 = local write "seqMsg"(w399) -> ()
        n198 = Subtract(x=w405, y=w406) -> (x-y=w402:u32)
        n199 = Less Than 0?(x=w402) -> (x < 0?=w403:bool)
        n200 = Select(t=u32 0, s=w403, f=w402) -> (s? t:f=w400:u32)
        n201 = Initialize Array(w400, 1 ("dimension size")) -> (w407:u32[])
        n202 = property on="seqMsg" class="Arr (strict)"("Index Values"=w407) -> ()  [unwired: 2 in, 2 out]
      }
      frame 4 {
      }
    }
  }
  n203 = flat-sequence {
    tunnel: w4 -> [w419]
    tunnel: w14 -> [_]
    frame #0 {
      n204 = Delete Data Value Reference(data value reference=w419) -> ()  [unwired: 1 in, 2 out]
    }
  }
